vi "Set XY Cluster.vi"(8 "Color":u32(colorbox), 9 "Y":i16, 10 "X":i16, 11 "Point In":refnum<class "Point.lvclass">) -> (3 "Point Out":refnum<class "Point.lvclass">)   [LabVIEW 2023, in "Point.lvclass"]
doc: "Set the X coordinate, Y coordinate, and color of the point."
uses:
  Point.lvclass
  c:/dev/_r/4/eng/lv-core/lvpostprocessingd/lv_mc_x86_64/dist_i386/examples/Object-Oriented Programming/Graphics/Graphic/Graphic.lvclass
  Point.lvclass/Point.ctl
  Graphic/Graphic.lvclass
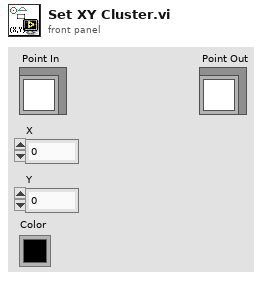
[diagram p1: front panel]
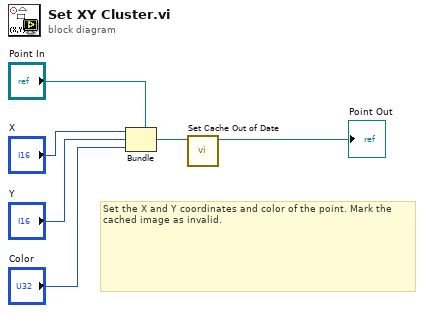
[diagram p0: block diagram]
diagram:
  # "Set the X and Y coordinates and color of the point. Mark the cached image as invalid."
  n1 = Bundle(cluster="Point In", "X", "Y", "Color") -> (w2:refnum<class "Point.lvclass">)
  n2 = call "Set Cache Out of Date.vi"("Graphic.lvclass"=w2) -> ("Graphic.lvclass out"=→"Point Out":refnum<class "Point.lvclass">)  [unwired: 10 in]
